vi "Init FIFO.vi"(8 "error in (no error)":errorcluster, 10 "Custom Config Data":u8[](array[numeric]), 11 "CIFfifo in":refnum<class "CIFfifo.lvclass">) -> (0 "error out":errorcluster, 2 "Depth":u64, 3 "CIFfifo out":refnum<class "CIFfifo.lvclass">)   [LabVIEW 2021, in "CIFfifo.lvclass"]
uses:
  CIFfifo.lvclass
  typedef/FIFO Header.ctl
  CIFfifo.lvclass/CIFfifo.ctl
  Accessors/Write Header.vi
  Accessors/Write Flags.vi
  Accessors/Write Buffer.vi
  <vilib>/CIF Foundation/CIF Utilities/DataTypes/Unflatten U64.vi
  Utilities/Expand FIFO Flags.vi
  ChannelCommon.lvlib
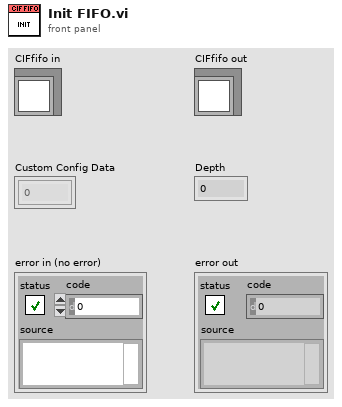
[diagram p1: front panel]
types:
  T1 = typedef "ChannelCommon.lvlib/FIFO Header.ctl" = cluster{"Length":u64, "T0":i64, "T_Out":i64, "T_Tx":i64, "Ctr":u64, "ClockID":u8}
  T2 = typedef "ChannelCommon.lvlib/FIFO Config.ctl" = cluster{"Max Bytes/Msg":u64, "Msg Depth":u64, "Flags":u64}
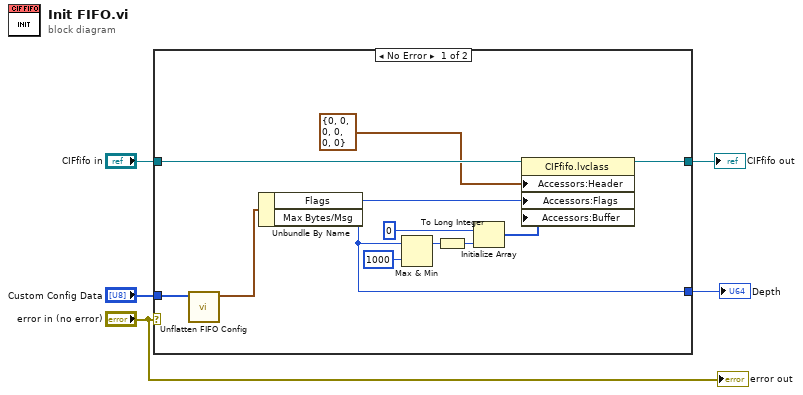
[diagram p0: block diagram]
diagram:
  n1 = case shown="No Error" "error in (no error)" {
    tunnel: [w16 w18] -> w4
    tunnel: "CIFfifo in" -> [w15 w18]
    tunnel: "Custom Config Data" -> [w6 _]
    tunnel: [w9 _] -> w2
    frame No Error {
      n2 = call "Unflatten FIFO Config.vi"("Flattened Data in"=w6) -> ("FIFO Config out"=w17:T2)  [unwired: 9 in, 1 out]
      n3 = Unbundle By Name(w17) -> ("Flags"=w14:u64, "Max Bytes/Msg"=w9:u64)
      n4 = Max & Min(x=w9, y=u64 1000) -> (max(x,y)=w8:u64)  [unwired: 1 out]
      n5 = To Long Integer(number=w8) -> (32bit integer=w10:i32)
      n6 = Initialize Array(u8 0, w10) -> (w12:u8[])
      n7 = property class="CIFfifo.lvclass"(reference=w15, "Accessors:Header"=T1 {"Length"=0, "T0"=0, "T_Out"=0, "T_Tx"=0, "Ctr"=0, "ClockID"=0} ("Header"), "Accessors:Flags"=w14, "Accessors:Buffer"=w12) -> (reference out=w16:refnum<class "CIFfifo.lvclass">)  [unwired: 1 in, 1 out]
    }
    frame Error {
    }
  }
  "CIFfifo out" <- w4
  "Depth" <- w2
  "error out" <- "error in (no error)"
